vi "WriteDataToQueueCMD.vi"(8 "error in (no error)":errorcluster, 10 "DataIn":string, 11 "ParameterConf in":refnum<class "ParameterConf.lvclass">) -> (0 "error out":errorcluster, 3 "ParameterConf out":refnum<class "ParameterConf.lvclass">)   [LabVIEW 2014, in "LibraryGcode.lvlib" / "ParameterConf.lvclass"]
uses:
  ParameterConf.lvclass
  ParameterConf.lvclass/ParameterConf.ctl
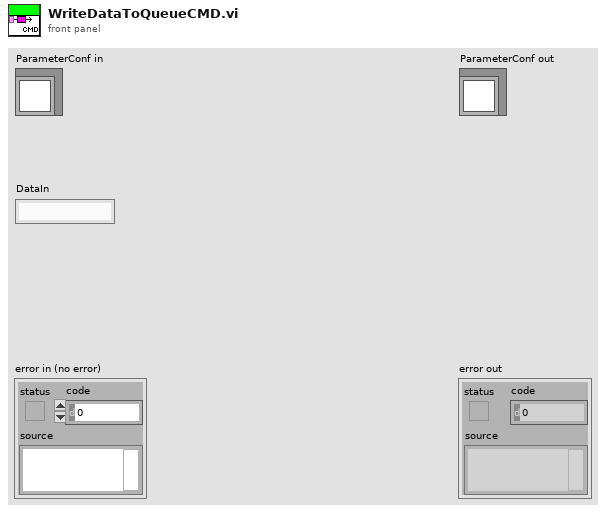
[diagram p1: front panel]
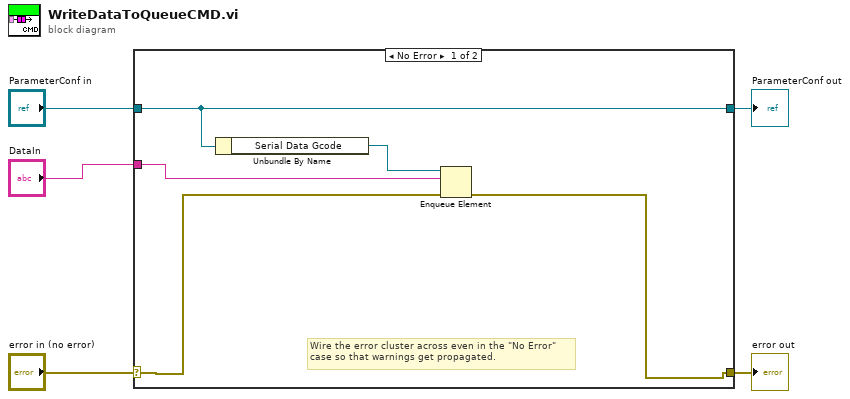
[diagram p0: block diagram]
diagram:
  n1 = case shown="No Error" "error in (no error)" {
    selector: "error in (no error)" -> [w7 w12]
    tunnel: [w6 w12] -> w4
    tunnel: [w10 w11] -> w2
    tunnel: "ParameterConf in" -> [w10 w11]
    tunnel: "DataIn" -> [w8 _]
    frame No Error {
      # "Wire the error cluster across even in the \"No Error\"\ncase so that warnings get propagated."
      n2 = Unbundle By Name(w10) -> ("Serial Data Gcode"=w9:refnum<queue>)
      n3 = Enqueue Element(queue=w9, element=w8, error in (no error)=w7) -> (error out=w6:errorcluster)  [unwired: 1 in, 2 out]
    }
    frame Error {
    }
  }
  "error out" <- w4
  "ParameterConf out" <- w2
